vi "Shooter Controller.vi"(8 "error in":errorcluster) -> ()   [LabVIEW 2020]
doc: "This VI executes continuously carrying out the current operation and responding to updates or new operations. It will often contain the timing or control code that is difficult to place directly in TeleOp. This VI generally opens all sensors and motors and isolates the rest of the robot code from knowing how the operations are carried out."
uses:
  <vilib>/Rock Robotics/WPI/Framework/Completion Status.ctl
  Shooter Setpoints.ctl
  Shooter Operations.ctl
  <vilib>/Rock Robotics/WPI/SafetyOutput/WPI_SafetyOutputConfigMenu.ctl
  <vilib>/Rock Robotics/Network Tables/NT Write Number.vi
panel:
  in  "Interactive Values":T1
  out "Current\nCmd":string
  in  "Buttons":cluster{"Execute Cmd":bool, "Abort Cmd":bool}
  out "Command Timing":cluster{"Start Time (ms)":u32, "Iterations":i32}
  out "Status":T3
  # "Tip: It may be helpful to observe inputs and sensor values.\nYou may also want to display tuning or debugging controls."
  # "Interactive Command: You may fill in the settings for a command\nand schedule it with the Execute button. You can observe and abort\nany command while fine tuning the code for the controller."
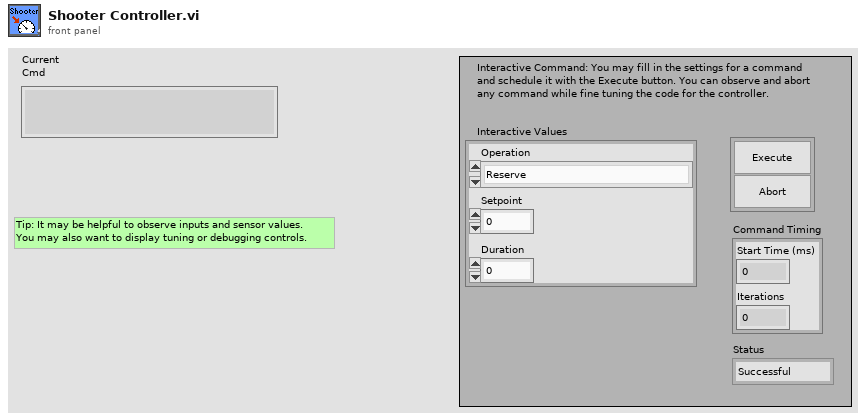
[diagram p1: front panel]
types:
  T1 = typedef "Shooter Setpoints.ctl" = cluster{"Operation":T2, "Setpoint":dbl, "Duration":dbl}
  T2 = typedef "Shooter Operations.ctl" = enum16{"Reserve", "Read Current", "Immediate", "with Duration", "Stop"}
  T3 = typedef "Completion Status.ctl" = enum16{"Successful", "Aborted", "Incomplete"}
  T4 = typedef "WPI_SafetyOutputConfigMenu.ctl" = enum16{"Enable", "Disable"}
  T5 = typedef "WPI_MotorControlDeviceRef.ctl" = cluster{"DeviceStatus":errorcluster, "Type":T6, "PWM":cluster{"PWM Channel":T7, "DeadBand":T8}, "CAN":cluster{"Device Number":u8, "SetOutput VI Ref":variant, "GetOutput VI Ref":variant, "Enable VI Ref":variant, "Disable VI Ref":variant, "Data":variant}, "Invert":bool, "DIO PWM":cluster{"PWM \"Enable\" Channel":T7, "DIOChannel":T9, "PWM Rate":dbl}}
  T6 = typedef "WPI_MotorControlType.ctl" = enum16{"PWM", "CAN", "DIO PWM"}
  T7 = typedef "FPGA_DIOPWMChannel.ctl" = enum8{"PWM 0", "PWM 1", "PWM 2", "PWM 3", "PWM 4", "PWM 5", "PWM 6", "PWM 7", "PWM 8", "PWM 9", "PWM MXP 0", "PWM MXP 1", "PWM MXP 2", "PWM MXP 3", "PWM MXP 4", "PWM MXP 5", "PWM MXP 6", "PWM MXP 7", "PWM MXP 8", "PWM MXP 9", "Invalid"}
  T8 = typedef "WPI_PWMDeadband.ctl" = cluster{"Name":string, "maxPositivePwm":i32, "minPositivePwm":i32, "centerPwm":i32, "maxNegativePwm":i32, "minNegativePwm":i32, "angularRange":u16}
  T9 = typedef "FPGA_DIOChannel.ctl" = enum8{"DIO 0", "DIO 1", "DIO 2", "DIO 3", "DIO 4", "DIO 5", "DIO 6", "DIO 7", "DIO 8", "DIO 9", "DIO MXP 0", "DIO MXP 1", "DIO MXP 2", "DIO MXP 3", "DIO MXP 4", "DIO MXP 5", "DIO MXP 6", "DIO MXP 7", "DIO MXP 8", "DIO MXP 9", "DIO MXP 10", "DIO MXP 11", "DIO MXP 12", "DIO MXP 13", "DIO MXP 14", "DIO MXP 15", "SPI Port CS1", "SPI Port CS2", "SPI Port CS3", "SPI Port MISO", "SPI Port MOSI", "Invalid"}
  T10 = typedef "Command Status Info.ctl" = cluster{"Name":string, "Status":T3, "notifier out":T11}
  T11 = typedef "Completion Notifier.ctl" = refnum<notifier>
  T12 = cluster{"Current Command":T1, "Command Timing":cluster{"Start Time (ms)":u32, "Iterations":i32}, "Command Arguments":cluster{"Command Info":T10, "Description":string, "Default Command":T1, "queue out":refnum<queue>, "Subsystem Name":string}}
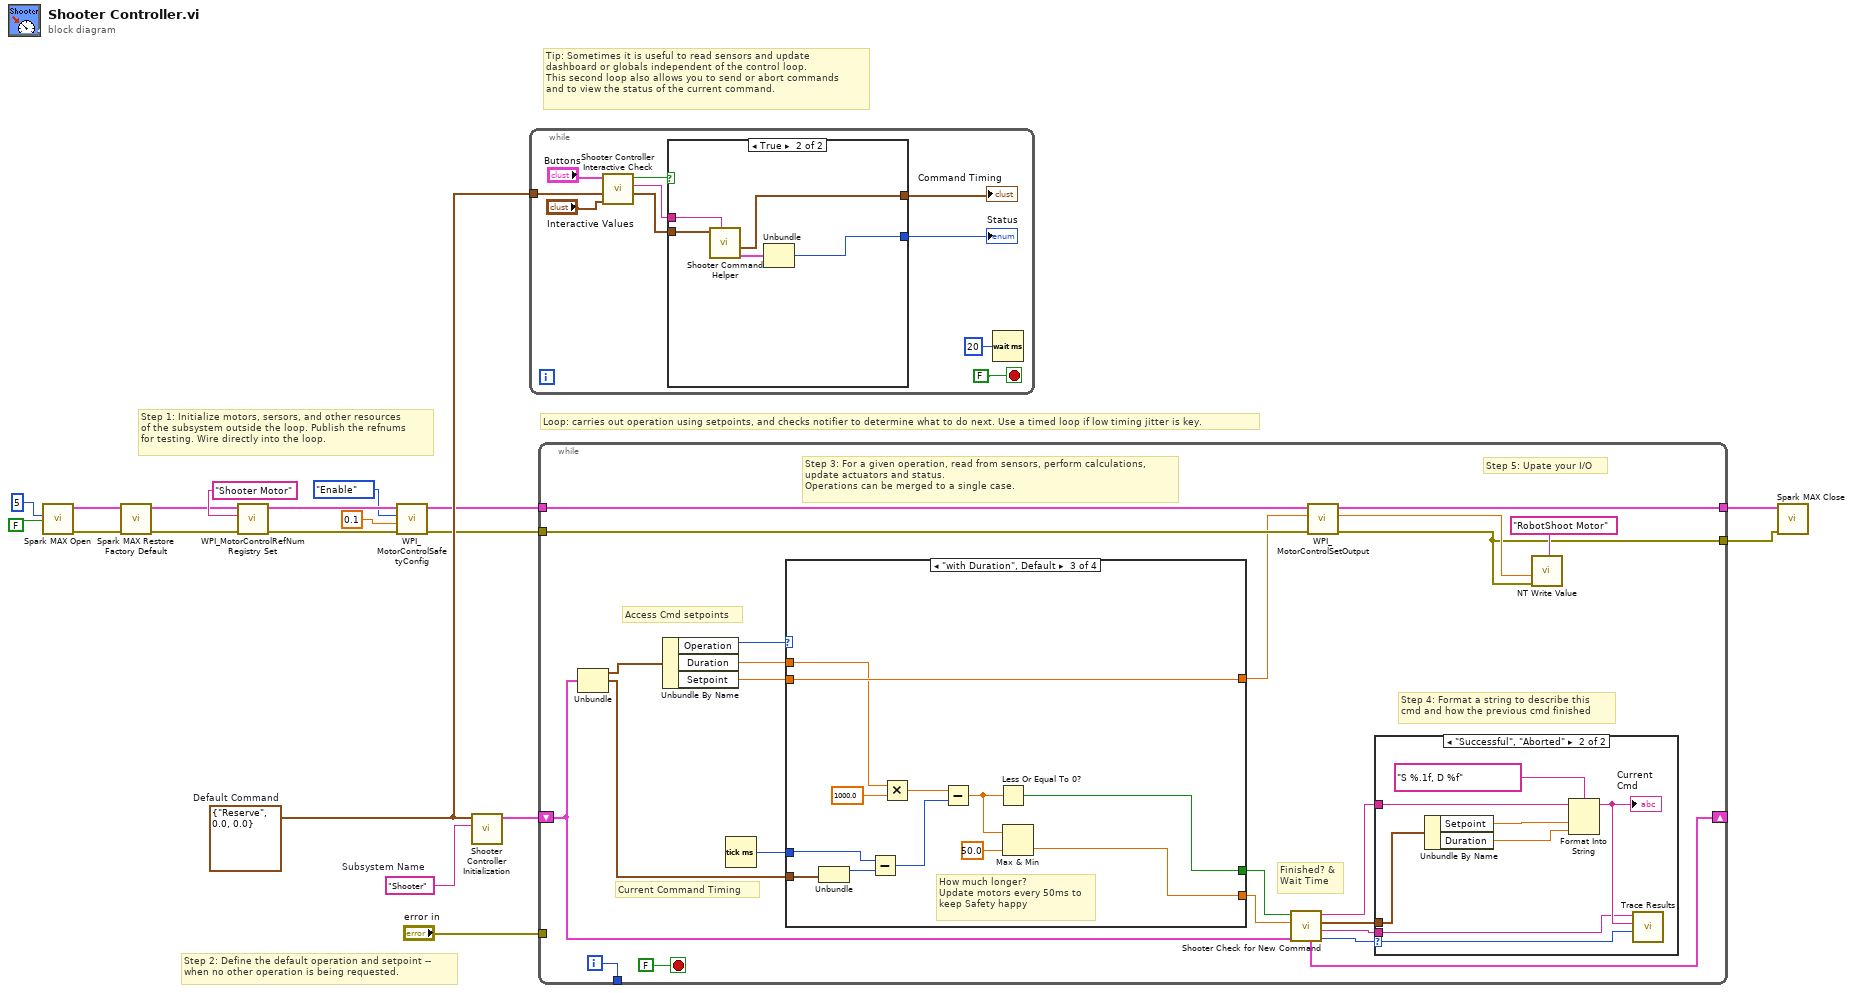
[diagram p0: block diagram]
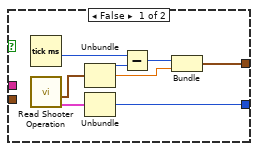
[diagram p2: hidden frame]
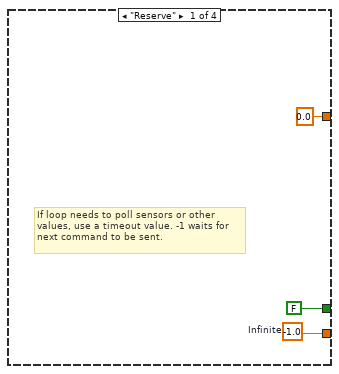
[diagram p4: hidden frame]
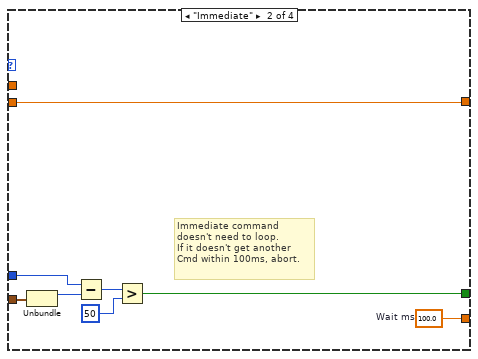
[diagram p5: hidden frame]
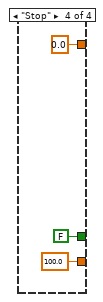
[diagram p6: hidden frame]
diagram:
  w16 = T1 {"Operation"=enum."Reserve", "Setpoint"=0.0, "Duration"=0.0}  # Default Command
  w17 = "Shooter"  # Subsystem Name
  # "Tip: Sometimes it is useful to read sensors and update\ndashboard or globals independent of the control loop.\nThis second loop also allows you to send or abort commands\nand to view the status of the current command."
  # "Step 2: Define the default operation and setpoint --\nwhen no other operation is being requested."
  # "Step 1: Initialize motors, sersors, and other resources\nof the subsystem outside the loop. Publish the refnums\nfor testing. Wire directly into the loop."
  # "Loop: carries out operation using setpoints, and checks notifier to determine what to do next. Use a timed loop if low timing jitter is key."
  n1 = call <vilib>:"Spark MAX Open.vi"("Invert"=FALSE, "Device Number"=u8 5) -> ("error out"=w6:errorcluster, "MotorControlDeviceRef"=w8:T5)  [unwired: 8 in]
  n2 = call <vilib>:"Spark MAX Restore Factory Default.vi"("error in"=w6, "MotorControlDeviceRef"=w8) -> ("error out"=w5:errorcluster, "MotorControlDeviceRef"=w7:T5)  [unwired: 8 in]
  n3 = call <vilib>:"WPI_MotorControlRefNum Registry Set.vi"("error in (no error)"=w5, "refnum name"="Shooter Motor", "MotorControlDevRef"=w7) -> ("error out"=w15:errorcluster, "MotorControlDevRef"=w14:T5)  [unwired: 7 in]
  n4 = call <vilib>:"WPI_MotorControlSafetyConfig.vi"("error in (no error)"=w15, "timeout (s)"=0.1, "mode"=WPI_SafetyOutputConfigMenu."Enable", "MotorControlDevRef"=w14) -> ("error out"=w2:errorcluster, "MotorControlDevRef"=w4:T5)  [unwired: 6 in]
  n5 = call "Shooter Controller Initialization.vi"("Subsystem Name"=w17, "Default Command"=w16) -> ("Current Command"=w18:T12)  [unwired: 9 in]
  n6 = while {
    tunnel: w16 -> [w26]
    stop <- FALSE stop-if-true
    n7 = call "Shooter Controller Interactive Check.vi"("Interactive Command in"="Interactive Values", "Default Command"=w26, "Buttons"="Buttons") -> ("Interactive Command out"=w23:T1, "Trace String"=w24:string, "Schedule"=w25:bool)  [unwired: 6 in]
    n8 = case shown="True" w25 {
      tunnel: [w37 w42] -> w22
      tunnel: w23 -> [_ w40]
      tunnel: [w33 w38] -> w21
      tunnel: w24 -> [_ w41]
      frame False {
        n9 = Tick Count (ms)() -> (millisecond timer value=w32:u32)
        n10 = call "Read Shooter Operation.vi"() -> ("Command Info"=w30:T10, "SubSystem Data"=w31:T1)  [unwired: 9 in, 1 out]
        n11 = Unbundle(w31) -> ("Operation"=w36:T2, "Setpoint"=w34:dbl)  [unwired: 1 out]
        n12 = Unbundle(w30) -> ("Status"=w37:T3)  [unwired: 2 out]
        n13 = Subtract(x=w32, y=w36) -> (x-y=w35:u32)
        n14 = Bundle(w35, "Setpoint"=w34) -> (w33:cluster{u32, "Setpoint":dbl})  [unwired: 1 in]
      }
      frame True {
        n15 = call "Shooter Command Helper.vi"("Description"=w41, "SubSystem Data"=w40) -> ("Command Info Out"=w39:T10, "Command Timing"=w38:cluster{"Start Time (ms)":u32, "Iterations":i32})  [unwired: 7 in, 1 out]
        n16 = Unbundle(w39) -> ("Status"=w42:T3)  [unwired: 2 out]
      }
    }
    "Status" <- w22
    "Command Timing" <- w21
    n17 = Wait (ms)(milliseconds to wait=u32 20) -> ()  [unwired: 1 out]
  }
  n18 = while {
    shift-right: [w57] -> _
    shift-left: w18 -> [w50]
    tunnel: [w64] -> _
    tunnel: "error in" -> [_]
    tunnel: w4 -> [w49]
    tunnel: [w48] -> w3
    tunnel: w2 -> [w47]
    tunnel: [w43] -> w1
    i -> [w64]
    stop <- FALSE stop-if-true
    # "Step 5: Upate your I/O"
    # "Step 4: Format a string to describe this\ncmd and how the previous cmd finished"
    # "Current Command Timing"
    # "Access Cmd setpoints"
    # "Finished? &\nWait Time"
    # "Step 3: For a given operation, read from sensors, perform calculations,\nupdate actuators and status.\nOperations can be merged to a single case."
    n19 = Unbundle(w50) -> ("Current Command"=w63:T1, "Command Timing"=w59:cluster{"Start Time (ms)":u32, "Iterations":i32})  [unwired: 1 out]
    n20 = Unbundle By Name(w63) -> ("Operation"=w62:T2, "Duration"=w61:dbl, "Setpoint"=w58:dbl)
    n21 = Tick Count (ms)() -> (millisecond timer value=w60:u32)
    n22 = case shown="\"with Duration\", Default" w62 {
      tunnel: [w76 w84 w87 100.0 ("Infinite")] -> w55
      tunnel: [FALSE ("ignore previous (F)") w78 w88 FALSE ("ignore previous (F)")] -> w56
      tunnel: w59 -> [_ w80 w90 _]
      tunnel: w61 -> [_ _ w85 _]
      tunnel: w60 -> [_ w79 w89 _]
      tunnel: w58 -> [_ w77 w86 _]
      tunnel: [0.0 ("Setpoint") w77 w86 0.0 ("Setpoint")] -> w46
      frame "Reserve" {
        w76 = -1.0  # Infinite
        # "If loop needs to poll sensors or other\nvalues, use a timeout value. -1 waits for\nnext command to be sent."
      }
      frame "Immediate" {
        w84 = 100.0  # Wait ms
        # "Immediate command\ndoesn't need to loop.\nIf it doesn't get another\nCmd within 100ms, abort."
        n23 = Unbundle(w80) -> ("Start Time (ms)"=w83:u32)  [unwired: 1 out]
        n24 = Subtract(x=w79, y=w83) -> (x-y=w82:u32)
        n25 = Greater?(x=w82, y=u8 50 ("Left Motor")) -> (0:w78:bool)
      }
      frame "with Duration", Default {
        # "How much longer?\nUpdate motors every 50ms to\nkeep Safety happy"
        n26 = Unbundle(w90) -> ("Start Time (ms)"=w95:u32)  [unwired: 1 out]
        n27 = Subtract(x=w89, y=w95) -> (x-y=w93:u32)
        n28 = Multiply(x=w85, y=1000.0) -> (x*y=w94:dbl)
        n29 = Subtract(x=w94, y=w93) -> (x-y=w96:dbl)
        n30 = Less Or Equal To 0?(x=w96) -> (x <= 0?=w88:bool)
        n31 = Max & Min(x=w96, y=50.0) -> (min(x,y)=w87:dbl)  [unwired: 1 out]
      }
      frame "Stop" {
      }
    }
    n32 = call "Shooter Check for New Command.vi"("Current Command"=w50, "Wait time (ms)"=w55, "Finished?"=w56) -> ("Completion"=w51:T3, "Subsystem Name"=w52:string, "Current Command"=w53:T1, "Initial Trace String"=w54:string, "NextCommand"=w57:T12)  [unwired: 4 in]
    n33 = call <vilib>:"WPI_MotorControlSetOutput.vi"("error in (no error)"=w47, "Output"=w46, "MotorControlDevRef"=w49) -> ("error out"=w43:errorcluster, "Motor Output"=w45:dbl, "MotorControlDevRef"=w48:T5)  [unwired: 6 in]
    n34 = case shown="\"Successful\", \"Aborted\"" w51 {
      selector: w51 -> [_ w73]
      tunnel: w54 -> [_ w69]
      tunnel: w53 -> [_ w70]
      tunnel: w52 -> [_ w66]
      frame "Incomplete", Default {
        # "Continuing current command"
      }
      frame "Successful", "Aborted" {
        # "Report and setup for next command"
        n35 = Unbundle By Name(w70) -> ("Setpoint"=w72:dbl, "Duration"=w67:dbl)
        n36 = Format Into String(format string="S %.1f, D %f", initial string=w69, w72, w67) -> (resulting string=w68:string)  [unwired: 1 in, 1 out]
        "Current\nCmd" <- w68
        n37 = call <vilib>:"Trace Results.vi"("Status of previous command"=w73, "Description"=w68, "Subsystem"=w66) -> ()  [unwired: 9 in]
      }
    }
    n38 = call-poly <vilib>:"NT Write Value.vi"("error in"=w43, "Numeric"=w45, "Name"="RobotShoot Motor") -> ()  [unwired: 8 in, 1 out]
  }
  n39 = call <vilib>:"Spark MAX Close.vi"("error in"=w1, "MotorControlDeviceRef"=w3) -> ()  [unwired: 9 in, 1 out]
